vi "subAcquisition_UpdateXY.vi"(6 "Grid step size (mm)":dbl[](array[numeric])=[0.22186666666666666, 0.22186666666666666], 7 "Stage Status Ref":refnum<vi>, 8 "error in":errorcluster, 9 "Yj":i32, 10 "Xi":i32, 11 "XY tiling":T1={"Tiling?"=FALSE, "YY/XX"=[1, 1], "X0Y0"=[-1.0, -12.0, 0.0]}) -> (0 "error out":errorcluster)   [LabVIEW 2015]
panel:
  # "X"
  # "Y"
  # "X"
  # "Y"
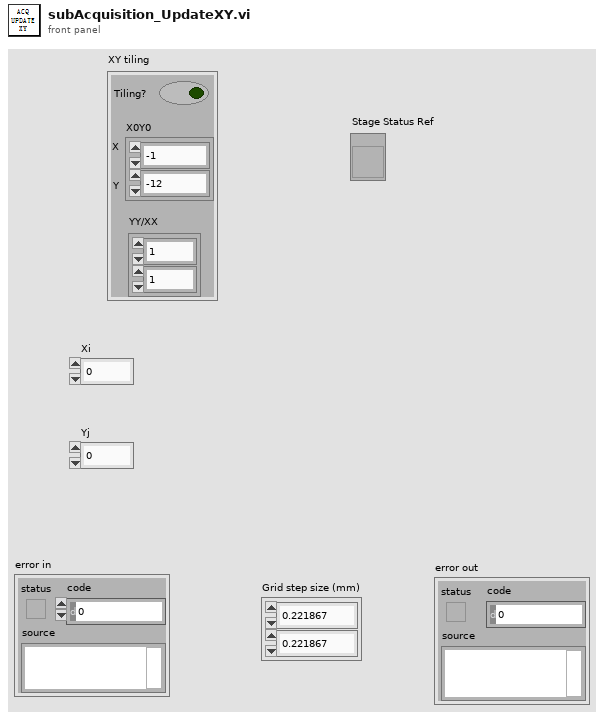
[diagram p1: front panel]
types:
  T1 = cluster{"Tiling?":bool, "YY/XX":i32[], "X0Y0":dbl[]}
  T2 = cluster{" Current Position":dbl[], "Number of Axis":i32, "ILSID":i32}
  T3 = cluster{"Console":cluster{"L":bool, "R":bool, "FWD":bool, "BACK":bool}, "Step Width [mm]":dbl, "Destination [mm]":dbl[], "Move ":bool}
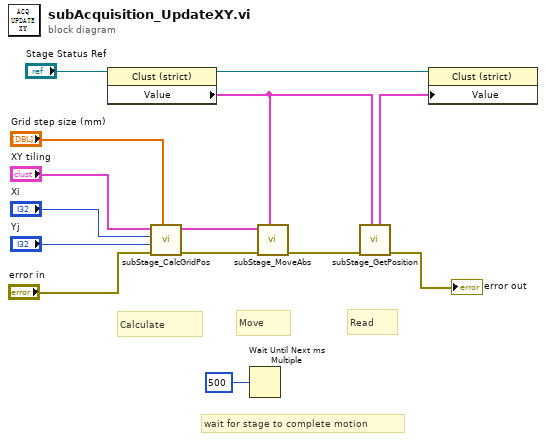
[diagram p0: block diagram]
diagram:
  # "Read"
  # "Move"
  # "Calculate"
  # "wait for stage to complete motion"
  n1 = property class="Clust (strict)"(reference="Stage Status Ref") -> (reference out=w1:refnum<vi>, "Value"=w3:T2)  [unwired: 1 in, 1 out]
  n2 = call "subStage_CalcGridPos.vi"("Grid step size (mm)"="Grid step size (mm)", "error in (no error)"="error in", "Yj"="Yj", "Xi"="Xi", "XY scan"="XY tiling") -> ("error out"=w14:errorcluster, "Stage-Ctrl"=w6:T3)  [unwired: 5 in]
  n3 = Wait Until Next ms Multiple(millisecond multiple=u32 500) -> ()  [unwired: 1 out]
  n4 = call "subStage_MoveAbs.vi"("Stage Info"=w3, "error in (no error)"=w14, "Stage-Ctrl"=w6) -> ("error out"=w5:errorcluster)  [unwired: 8 in]
  n5 = call "subStage_GetPosition.vi"("Stage Info In"=w3, "Error In"=w5) -> ("Error out"=→"error out":errorcluster, "Stage Info Out"=w2:T2)  [unwired: 8 in]
  n6 = property class="Clust (strict)"(reference=w1, "Value"=w2) -> ()  [unwired: 1 in, 2 out]
